vi "RampTest.vi"() -> ()   [LabVIEW 2016]
doc: "The myRIO Project template acquires acceleration data from the onboard accelerometer and displays the changes of acceleration values in a waveform chart."
uses:
  Project Custom Controls/IMU Data Cluster.ctl
  <vilib>/Analysis/1siggen.llb/Ramp Pattern by Samples.vi
  <vilib>/myRIO/Common/Instrument Driver Framework/myRIO v1.0/UART/vis/myRIO v1.0 Close UART.vi
  <vilib>/Instr/_visa.llb/VISA Configure Serial Port (Instr).vi
  <vilib>/Utility/error.llb/Error Cluster From Error Code.vi
  <vilib>/myRIO/Common/Instrument Driver Framework/myRIO v1.0/PWM/vis/myRIO v1.0 Write PWM.vi
  <vilib>/myRIO/Common/Instrument Driver Framework/Utilities/vis/FPGA Ref Manager.vi
  <vilib>/myRIO/Common/Instrument Driver Framework/myRIO v1.0/myRIO v1.0 Reset FPGA.vi
  <vilib>/myRIO/Common/Instrument Driver Framework/myRIO v1.0/IRQ/vis/myRIO v1.0 IRQ Info FGV.vi
  <vilib>/myRIO/Common/Instrument Driver Framework/myRIO v1.0/IRQ/vis/myRIO v1.0 Timer IRQ Info FGV.vi
  <vilib>/myRIO/Common/Instrument Driver Framework/myRIO v1.0/IRQ/vis/myRIO v1.0 ISR Agent.vi
  <vilib>/myRIO/Instrument Drivers/Utilities/Utilities.lvlib
  <vilib>/myRIO/Instrument Drivers/Onboard IO/PWM/PWM.lvlib
  <vilib>/Analysis/NI_AALBase.lvlib
panel:
  out "PWM 2":dbl
  in  "Start 2":bool
  out "PWM":dbl
  in  "Yaw Gains 3":T1
  in  "Yaw 3":dbl min=0.0 max=0.08
  in  "Yaw Gains 2":T1
  in  "Yaw 2":dbl min=0.0 max=0.08
  in  "Start":bool
  out "Boolean 3":bool
  out "Boolean 2":bool
  out "Loop Iteration":dbl
  out "Waveform Chart":cluster{"Yaw":dbl, "Pitch":dbl, "Roll":dbl}(graph)
  in  "Stop":bool
  out "IMU Data Cluster":T2
  out "Boolean":bool
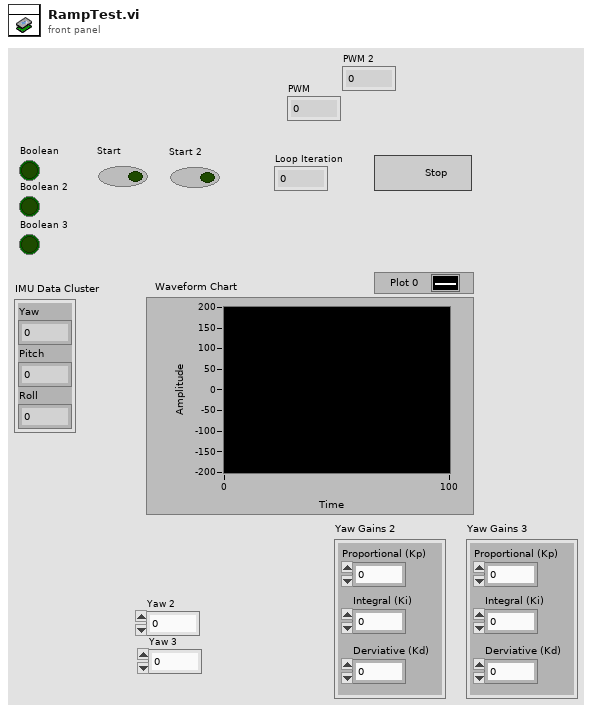
[diagram p1: front panel]
types:
  T1 = cluster{"Proportional (Kp)":dbl, "Integral (Ki)":dbl, "Derviative (Kd)":dbl}
  T2 = typedef "IMU Data Cluster.ctl" = cluster{"Yaw":dbl, "Pitch":dbl, "Roll":dbl}
  T3 = typedef "PWM.lvlib/PWM Reference.ctl" = cluster{"myRIO Reference":T4, "PWM Channels Enum":T8, "PWM Configuration":T9}
  T4 = typedef "myRIO Generic Hardware Reference.ctl" = cluster{"myRIO Model":T5, "myRIO Hardware Reference":T6}
  T5 = typedef "Hardware Version Enum.ctl" = enum16{"Unknown", "myRIO-1900", "myRIO-1950", "roboRIO", "NI ELVIS RIO CM"}
  T6 = typedef "myRIO v1.0 Reference.ctl" = cluster{"Generic FPGA Reference":T7, "Allow multiple opens":bool}
  T7 = typedef "Generic FPGA Reference.ctl" = refnum<k20>
  T8 = typedef "PWM Channels Enum.ctl" = enum16{"Not Connected", "C/PWM0", "C/PWM1", "A/PWM0", "A/PWM1", "A/PWM2", "B/PWM0", "B/PWM1", "B/PWM2", "PWM/PWM0", "PWM/PWM1", "PWM/PWM2", "PWM/PWM3", "PWM/PWM4", "PWM/PWM5", "PWM/PWM6", "PWM/PWM7", "PWM/PWM8", "PWM/PWM9"}
  T9 = typedef "PWM.lvlib/PWM Configuration.ctl" = cluster{"Frequency":dbl, "Duty Cycle":dbl}
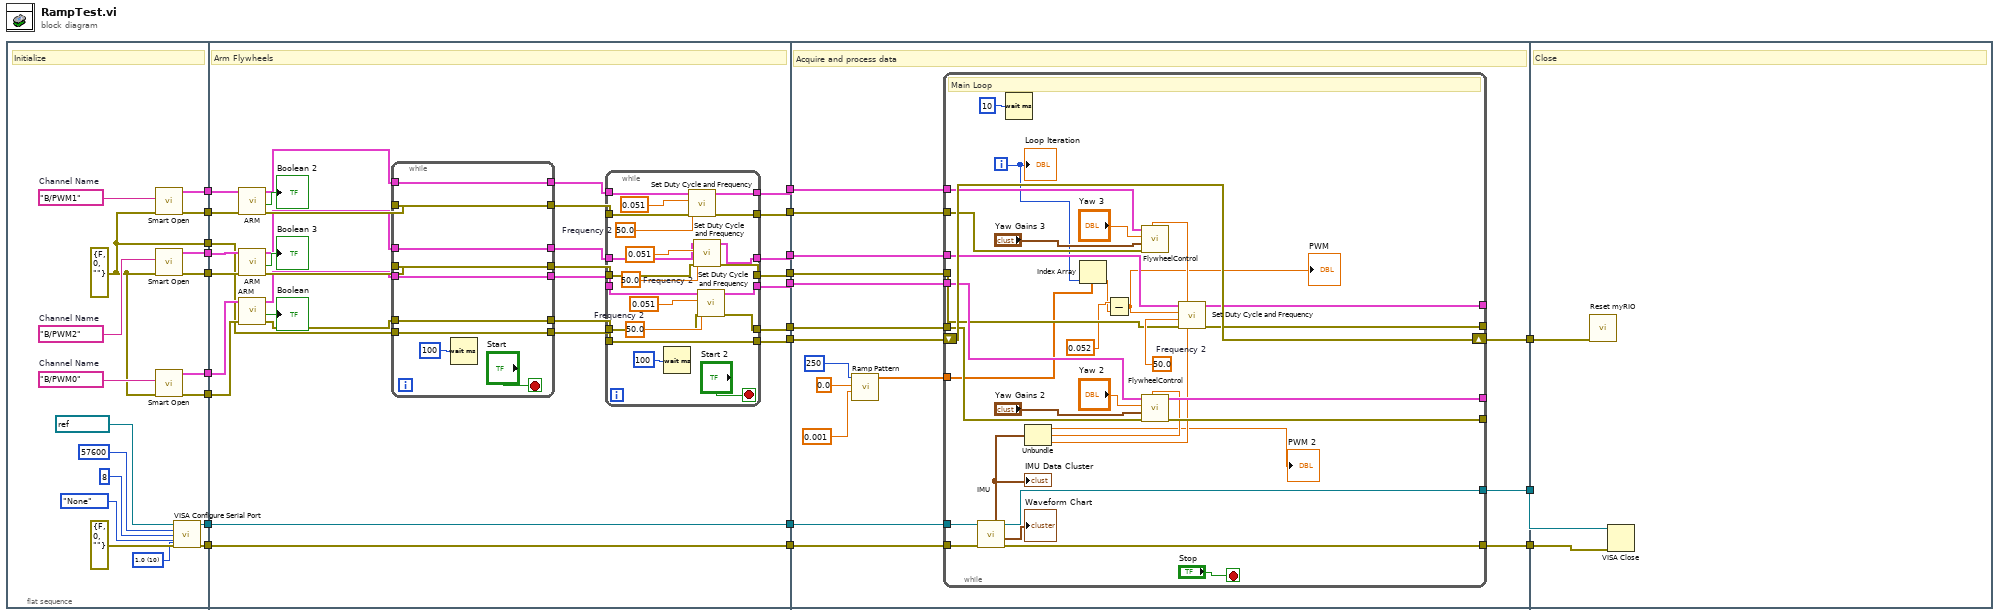
[diagram p0: block diagram]
diagram:
  n1 = flat-sequence {
    tunnel: [w34] -> w20
    tunnel: [w39] -> w19
    tunnel: [w38] -> w18
    tunnel: [w33] -> w17
    tunnel: [w32] -> w16
    tunnel: [w31] -> w15
    tunnel: [w30] -> w14
    tunnel: [w23] -> w5
    tunnel: [w22] -> w3
    tunnel: w20 -> [w62]
    tunnel: w19 -> [w71]
    tunnel: w18 -> [w70]
    tunnel: w17 -> [w69]
    tunnel: w16 -> [w68]
    tunnel: w15 -> [w67]
    tunnel: w14 -> [w66]
    tunnel: [w46] -> w13
    tunnel: [w45] -> w12
    tunnel: [w44] -> w11
    tunnel: [w43] -> w10
    tunnel: [w40] -> w9
    tunnel: [w41] -> w8
    tunnel: [w42] -> w7
    tunnel: [w55] -> w6
    tunnel: w5 -> [w55]
    tunnel: [w54] -> w4
    tunnel: w3 -> [w54]
    tunnel: [w117] -> w21
    tunnel: w13 -> [w116]
    tunnel: w12 -> [w115]
    tunnel: w11 -> [w114]
    tunnel: w10 -> [w113]
    tunnel: w9 -> [w110]
    tunnel: w8 -> [w112]
    tunnel: w7 -> [w111]
    tunnel: w6 -> [w108]
    tunnel: w4 -> [w109]
    tunnel: [w107] -> w2
    tunnel: [w106] -> w1
    tunnel: w21 -> [w152]
    tunnel: w2 -> [w151]
    tunnel: w1 -> [w150]
    frame #0 {
      w25 = u16 10 items=["1.0"=10, "1.5"=15, "2.0"=20] ("stop bits (10: 1 bit)")
      w35 = tag "B/PWM2"  # Channel Name
      w36 = tag "B/PWM1"  # Channel Name
      w37 = tag "B/PWM0"  # Channel Name
      w34 = errorcluster {"status"=FALSE, "code"=0, "source"=""} ("error in (no error)")
      # "Initialize"
      n2 = call <vilib>:"Smart Open.vi"("error in (no error)"=w34, "Channel Name"=w36) -> ("error out"=w32:errorcluster, "PWM Ref Out"=w33:T3)  [unwired: 8 in]
      n3 = call <vilib>:"Smart Open.vi"("error in (no error)"=w34, "Channel Name"=w35) -> ("error out"=w30:errorcluster, "PWM Ref Out"=w31:T3)  [unwired: 8 in]
      n4 = call <vilib>:"Smart Open.vi"("error in (no error)"=w34, "Channel Name"=w37) -> ("error out"=w38:errorcluster, "PWM Ref Out"=w39:T3)  [unwired: 8 in]
      n5 = call-poly "VISA Configure Serial Port"("VISA resource name"=refnum<visa-resource-name> "ASRL2::INSTR", "baud rate (9600)"=u32 57600, "data bits (8)"=u16 8, "parity (0:none)"=enum16{"None", "Odd", "Even", "Mark", "Space"}."None", "error in (no error)"=errorcluster {"status"=FALSE, "code"=0, "source"=""}, "stop bits (10: 1 bit)"=w25) -> ("VISA resource name out"=w23:refnum<visa-resource-name>, "error out"=w22:errorcluster)  [unwired: 8 in]
    }
    frame #1 {
      # "Arm Flywheels"
      n6 = call "ARM.vi"("error in (no error)"=w68, "PWM Ref in"=w69) -> ("error out"=w59:errorcluster, "Boolean"=→"Boolean 2":bool, "PWM Ref out"=w60:T3)  [unwired: 7 in]
      n7 = call "ARM.vi"("error in (no error)"=w66, "PWM Ref in"=w67) -> ("error out"=w57:errorcluster, "Boolean"=→"Boolean 3":bool, "PWM Ref out"=w58:T3)  [unwired: 7 in]
      n8 = call "ARM.vi"("error in (no error)"=w70, "PWM Ref in"=w71) -> ("error out"=w61:errorcluster, "Boolean"=→"Boolean":bool, "PWM Ref out"=w56:T3)  [unwired: 7 in]
      n9 = while {
        tunnel: w62 -> [w100]
        tunnel: [w100] -> w53
        tunnel: w61 -> [w98]
        tunnel: w60 -> [w93]
        tunnel: w59 -> [w94]
        tunnel: w58 -> [w95]
        tunnel: w57 -> [w96]
        tunnel: w56 -> [w97]
        tunnel: [w98] -> w52
        tunnel: [w97] -> w51
        tunnel: [w96] -> w50
        tunnel: [w95] -> w49
        tunnel: [w94] -> w48
        tunnel: [w93] -> w47
        stop <- "Start" stop-if-true
        n10 = Wait (ms)(milliseconds to wait=u32 100) -> ()  [unwired: 1 out]
      }
      n11 = while {
        tunnel: w53 -> [w91]
        tunnel: [w91] -> w40
        tunnel: [w82] -> w41
        tunnel: w52 -> [w83]
        tunnel: [w75] -> w46
        tunnel: w47 -> [w72]
        tunnel: [w74] -> w45
        tunnel: w48 -> [w73]
        tunnel: [w77] -> w44
        tunnel: w49 -> [w79]
        tunnel: [w76] -> w43
        tunnel: w50 -> [w78]
        tunnel: [w81] -> w42
        tunnel: w51 -> [w80]
        stop <- "Start 2" stop-if-true
        w85 = 50.0  # Frequency 2
        w87 = 50.0  # Frequency 2
        w89 = 50.0  # Frequency 2
        n12 = Wait (ms)(milliseconds to wait=u32 100) -> ()  [unwired: 1 out]
        n13 = call <vilib>:"Set Duty Cycle and Frequency.vi"("error in (no error)"=w73, "Frequency [Hz]"=w89, "Duty Cycle"=0.051 ("start"), "PWM Ref In"=w72) -> ("error out"=w74:errorcluster, "PWM Ref Out"=w75:T3)  [unwired: 5 in]
        n14 = call <vilib>:"Set Duty Cycle and Frequency.vi"("error in (no error)"=w78, "Frequency [Hz]"=w87, "Duty Cycle"=0.051 ("start"), "PWM Ref In"=w79) -> ("error out"=w76:errorcluster, "PWM Ref Out"=w77:T3)  [unwired: 5 in]
        n15 = call <vilib>:"Set Duty Cycle and Frequency.vi"("error in (no error)"=w83, "Frequency [Hz]"=w85, "Duty Cycle"=0.051 ("start"), "PWM Ref In"=w80) -> ("error out"=w82:errorcluster, "PWM Ref Out"=w81:T3)  [unwired: 5 in]
      }
    }
    frame #2 {
      # "Acquire and process data"
      n16 = call-poly <vilib>:"Ramp Pattern.vi"("start"=0.001, "end"=0.0, "samples"=250) -> ("Ramp Pattern"=w102:dbl[])  [unwired: 7 in, 1 out]
      n17 = while {
        shift-right: [w142] -> w117
        shift-left: w110 -> [w142]
        tunnel: w112 -> [w141]
        tunnel: w111 -> [w140]
        tunnel: w116 -> [w139]
        tunnel: w115 -> [w138]
        tunnel: w114 -> [w127]
        tunnel: w113 -> [w126]
        tunnel: w109 -> [w148]
        tunnel: w108 -> [w147]
        tunnel: [w146] -> w107
        tunnel: [w145] -> w106
        tunnel: [w135] -> _
        tunnel: [w134] -> _
        tunnel: [w124] -> _
        tunnel: [w123] -> _
        tunnel: w102 -> [w122]
        i -> [w125]
        stop <- "Stop" stop-if-true
        w128 = 50.0  # Frequency 2
        # "Main Loop"
        n18 = call "IMU.vi"("error in (no error)"=w148, "VISA Refnum in"=w147) -> ("error out"=w145:errorcluster, "Waveform Chart"=→"Waveform Chart":cluster{"Yaw":dbl, "Pitch":dbl, "Roll":dbl}, "VISA Refnum out"=w146:refnum<visa-resource-name>, "IMU Data Cluster"=w131:T2)  [unwired: 5 in, 1 out]
        "IMU Data Cluster" <- w131
        n19 = Wait (ms)(milliseconds to wait=u32 10) -> ()  [unwired: 1 out]
        n20 = Unbundle(w131) -> ("Yaw"=→"PWM 2":dbl, "Pitch"=w129:dbl, "Roll"=w130:dbl)
        n21 = Index Array(array=w122, index=w125) -> (element=w118:dbl)
        n22 = Subtract(x=0.052 ("start"), y=w118) -> (x-y=w120:dbl)
        "PWM" <- w120
        n23 = call "FlywheelControl.vi"("Numeric"=w130, "error in (no error)"=w138, "Yaw Gains"="Yaw Gains 3", "Yaw"="Yaw 3", "PWM Ref in"=w139) -> ()  [unwired: 5 in, 2 out]
        n24 = call "FlywheelControl.vi"("Numeric"=w129, "error in (no error)"=w141, "Yaw Gains"="Yaw Gains 2", "Yaw"="Yaw 2", "PWM Ref in"=w140) -> ("error out"=w134:errorcluster, "PWM Ref Out"=w135:T3)  [unwired: 5 in]
        n25 = call <vilib>:"Set Duty Cycle and Frequency.vi"("error in (no error)"=w126, "Frequency [Hz]"=w128, "Duty Cycle"=w120, "PWM Ref In"=w127) -> ("error out"=w123:errorcluster, "PWM Ref Out"=w124:T3)  [unwired: 5 in]
        "Loop Iteration" <- w125
      }
    }
    frame #3 {
      # "Close"
      n26 = call <vilib>:"Reset myRIO.vi"("error in (no error)"=w152) -> ()  [unwired: 10 in, 1 out]
      n27 = VISA Close(VISA resource name=w151, error in (no error)=w150) -> ()  [unwired: 1 out]
    }
  }
